vi "Read EventLog.vi"(8 "error in (no error)":errorcluster, 11 "bt_Log in":refnum<class "bt_Log.lvclass">) -> (0 "error out":errorcluster, 2 "abs_EventLog.lvclass":refnum<class "abs_EventLog.lvclass">, 3 "bt_Log out":refnum<class "bt_Log.lvclass">)   [LabVIEW 2021, in "BT.lvlib" / "bt_Log.lvclass"]
uses:
  bt_Log.lvclass
  <vilib>/TSA/Event Log/abs_EventLog/abs_EventLog.lvclass
  bt_Log.lvclass/bt_Log.ctl
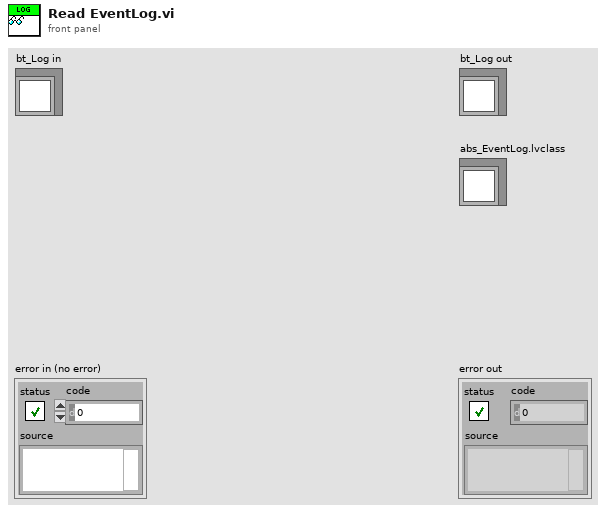
[diagram p1: front panel]
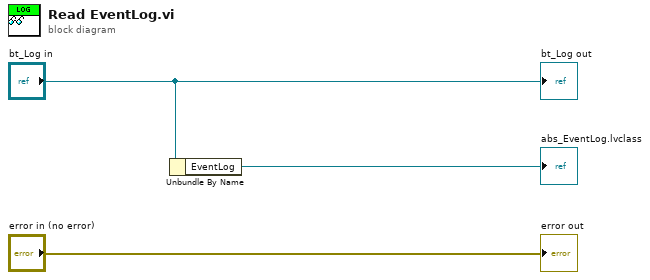
[diagram p0: block diagram]
diagram:
  n1 = Unbundle By Name("bt_Log in") -> ("EventLog"=→"abs_EventLog.lvclass":refnum<class "abs_EventLog.lvclass">)
  "error out" <- "error in (no error)"
  "bt_Log out" <- "bt_Log in"
